vi "06_dosing.vi"() -> ()   [LabVIEW 2024]
uses:
  <vilib>/Utility/error.llb/DialogType.ctl
  7567123a-d5c5-487a-bc91-47e086c159d1.vi
  <vilib>/Waveform/WDTOps.llb/WDT Waveform to XY Pairs DBL.vi
  <instrlib>/Tektronix DMM40x0 Series/Tektronix DMM40x0 Series.lvlib
panel:
  out "Numeric":i32
  out "Waveform Graph 2":dbl[](array[numeric])
  out "STABLE":bool
  in  "Serial Communication":T1={"Baud Rate"=9600, "Parity"=0, "Data Bits"=8, "Stop Bits"=10, "Flow Control"=0} {"Flow Control" items=["None", "XON/XOFF", "RTS/CTS", "XON/XOFF & RTS/CTS", "DTR/DSR", "XON/XOFF & DTR/DSR"]; "Stop Bits" items=["1.0"=10, "1.5"=15, "2.0"=20]; "Data Bits" items=["7"=7, "8"=8]; "Parity" items=["None", "Odd", "Even", "Mark", "Space"]; "Baud Rate" items=["300"=300, "600"=600, "1200"=1200, "2400"=2400, "4800"=4800, "9600"=9600, "19200"=19200]}
  in  "COM PORT (COM2)":refnum<visa-resource-name>
  out "Stability threshold":dbl format="%#_13g"
  out "Waveform Graph":dbl[](graph)
  # "Voltmeter Serial Configuration"
  # "DEFAULT SETTINGS:\n\nTimeout (10000 ms)\nTrigger Count (5000)\nSample Count (1)\n\n****DC VOLTAGE***"
  # "Voltmeter Stability"
  # "0 - Stability threshold not met\n1 - Stability threshold met\n\n\n\n*stability (+/-0.05 mV) of last 15 pts"
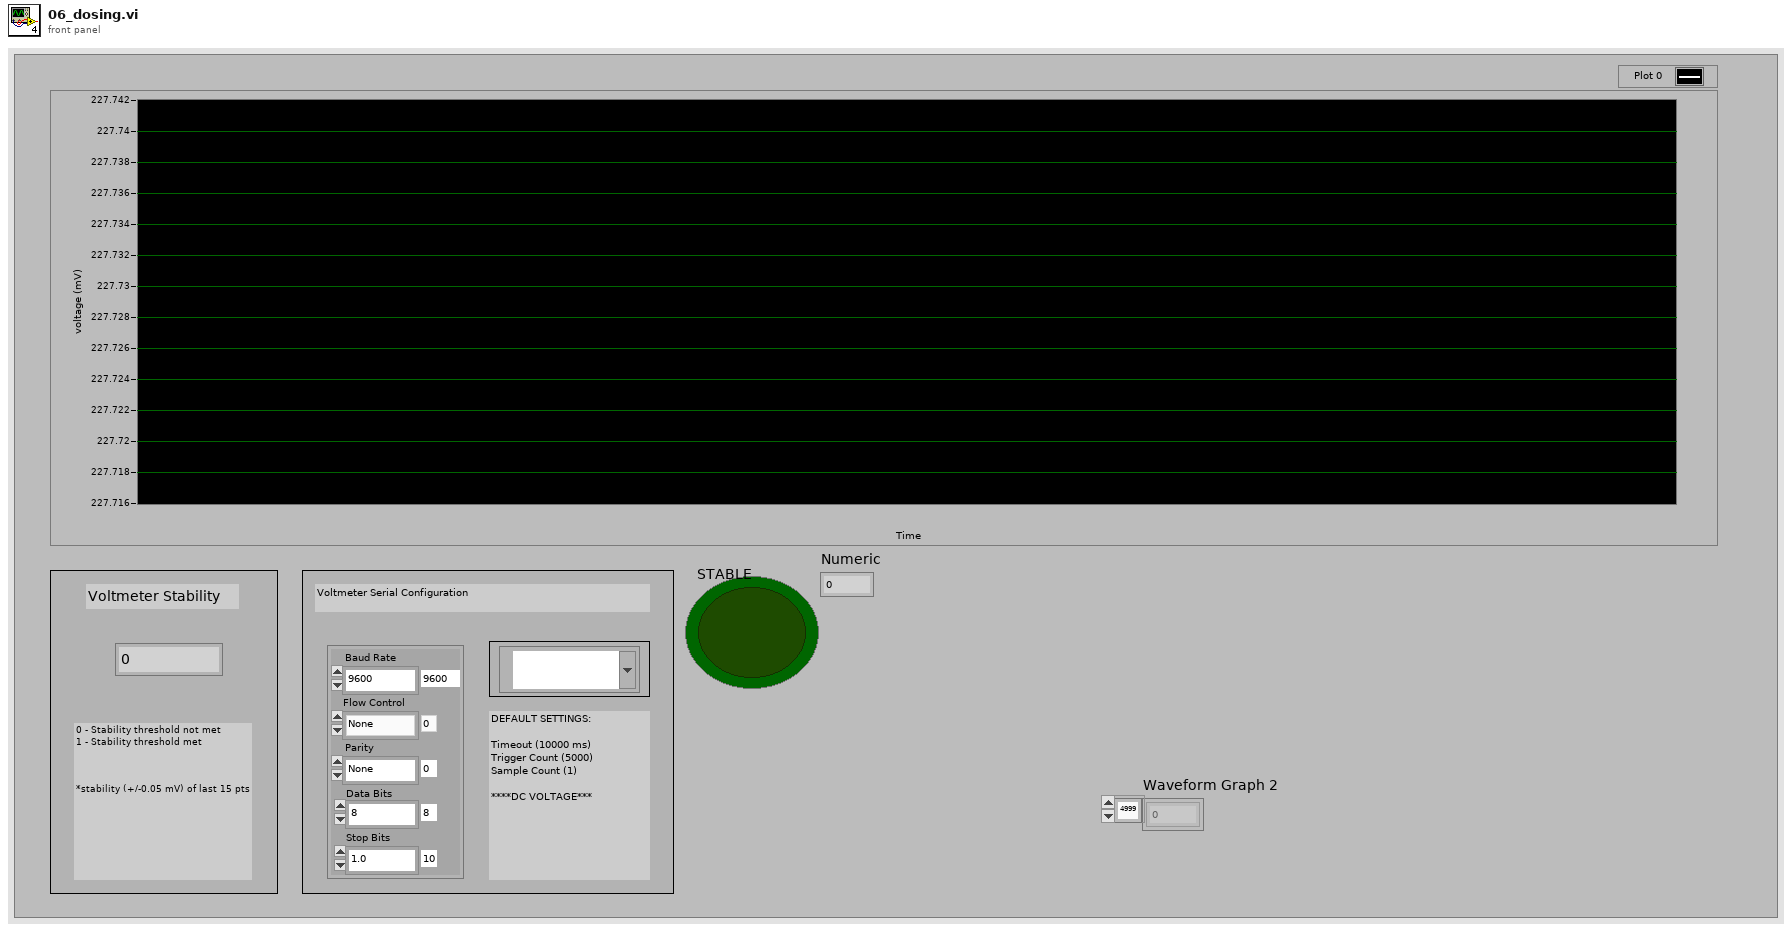
[diagram p1: front panel]
types:
  T1 = cluster{"Baud Rate":u32, "Parity":u16, "Data Bits":u16, "Stop Bits":u16, "Flow Control":u16}
  T2 = typedef "DialogType.ctl" = u16
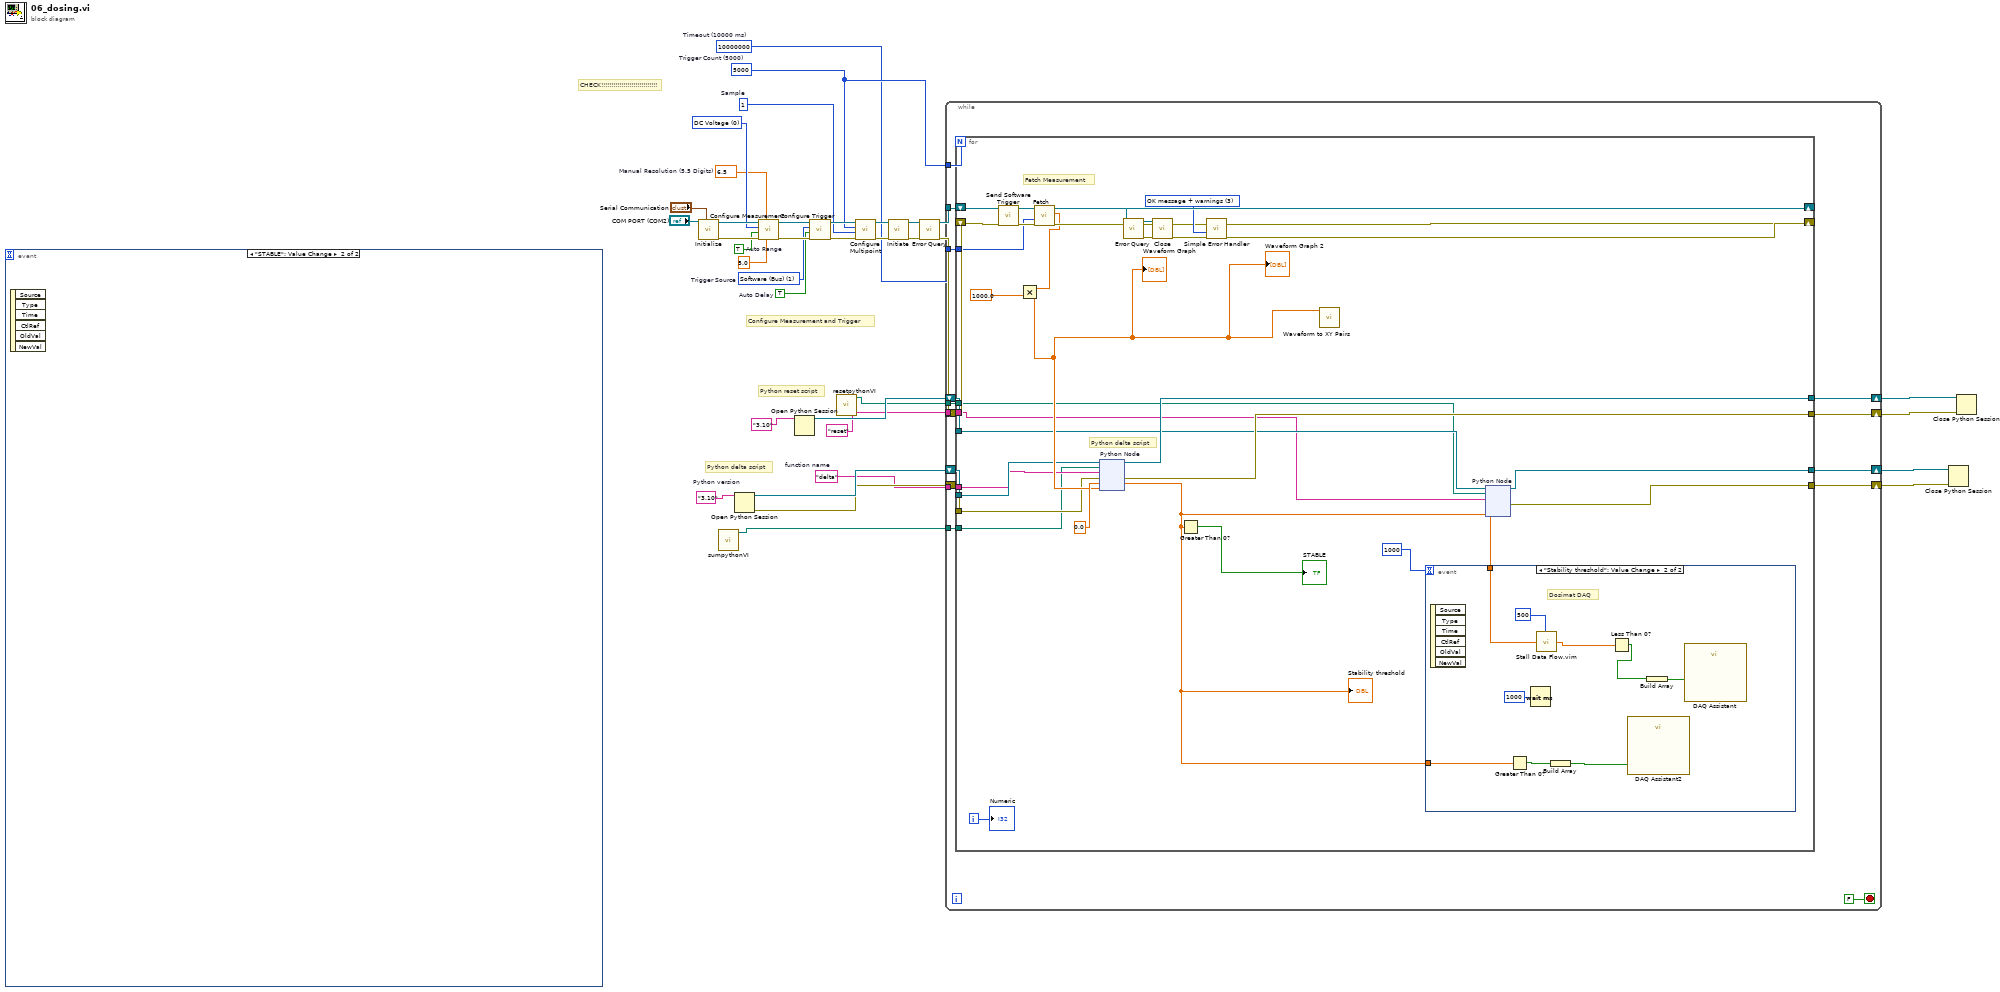
[diagram p0: block diagram]
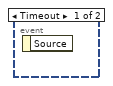
[diagram p2: hidden frame]
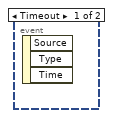
[diagram p3: hidden frame]
diagram:
  w8 = "delta"  # function name
  w11 = "3.10"  # Python version
  w23 = u16 0 items=["DC Voltage", "AC Voltage", "2 - Wire Resistance", "4 - Wire Resistance", "DC Current", "AC Current", "Frequency", "Period", "Continuity", "Diode Checking", "Temperature", "Capacitance"] ("Function (0: DC Voltage)")
  w14 = u32 10000000  # Timeout (10000 ms)
  w15 = 1  # Sample
  w22 = 5000  # Trigger Count (5000)
  w16 = 6.5 items=["4.5"=4.5, "5.5"=5.5, "6.5"=6.5]  # Manual Resolution (5.5 Digits)
  w24 = TRUE  # Auto Delay
  w25 = u16 1 items=["Immediate", "Software (Bus)", "External"]  # Trigger Source
  w26 = TRUE  # Auto Range
  # "Python delta script"
  # "Python reset script"
  # "CHECK!!!!!!!!!!!!!!!!!!!!!!!!!!!!"
  # "Configure Measurement and Trigger"
  n1 = event shown="[1] \"STABLE\": Value Change" {
    selector: _ -> [_ _]
    dyn-events: _ -> [_ _]
    timeout: _ -> [_ _]
    event Timeout {
      n2 = event-data() -> ()  [unwired: 1 in, 3 out]
    }
    event "STABLE": Value Change {
      n3 = event-data() -> ()  [unwired: 1 in, 6 out]
    }
  }
  n4 = call <instrlib>:"Initialize.vi"("Serial Configuration"="Serial Communication", "VISA resource name"="COM PORT (COM2)") -> ("error out"=w35:errorcluster, "VISA resource name out"=w36:refnum<visa-resource-name>)  [unwired: 3 in, 5 out]
  n5 = call "sumpythonVI.vi"() -> ("appended path"=w1:path)  [unwired: 11 in]
  n6 = Open Python Session(python version=w11) -> (session out=w13:refnum<k35>, error out=w12:errorcluster)  [unwired: 2 in]
  n7 = call <instrlib>:"Configure Measurement.vi"("Manual Range (1.0)"=5.0, "Manual Resolution (5.5 Digits)"=w16, "error in (no error)"=w35, "Auto Range (T:Enable)"=w26, "Function (0: DC Voltage)"=w23, "VISA resource name"=w36) -> ("error out"=w33:errorcluster, "VISA resource name out"=w34:refnum<visa-resource-name>)  [unwired: 4 out]
  n8 = Open Python Session(python version="3.10" ("Python version")) -> (session out=w9:refnum<k35>)  [unwired: 2 in, 1 out]
  n9 = call <instrlib>:"Configure Trigger.vi"("error in (no error)"=w33, "Auto Delay (T: Enable)"=w24, "Trigger Source (0: Immediate)"=w25, "VISA resource name"=w34) -> ("error out"=w31:errorcluster, "VISA resource name out"=w32:refnum<visa-resource-name>)  [unwired: 1 in, 5 out]
  n10 = call "resetpythonVI.vi"() -> ("appended path"=w7:path)  [unwired: 11 in]
  n11 = call <instrlib>:"Configure Multipoint.vi"("error in (no error)"=w31, "Sample Count (1)"=w15, "Trigger Count (1)"=w22, "VISA resource name"=w32) -> ("error out"=w29:errorcluster, "VISA resource name out"=w30:refnum<visa-resource-name>)  [unwired: 6 out]
  n12 = call <instrlib>:"Initiate.vi"("error in (no error)"=w29, "VISA resource name"=w30) -> ("error out"=w21:errorcluster, "VISA resource name out"=w20:refnum<visa-resource-name>)  [unwired: 8 out]
  n13 = call <instrlib>:"Error Query.vi"("error in (no error)"=w21, "VISA resource name"=w20) -> ("error out"=w18:errorcluster, "VISA resource name out"=w19:refnum<visa-resource-name>)  [unwired: 8 out]
  n14 = while {
    tunnel: w22 -> [w52]
    tunnel: w19 -> [w51]
    tunnel: w14 -> [w49]
    tunnel: w8 -> [w45]
    tunnel: w7 -> [w44]
    tunnel: "reset" ("function name") -> [w43]
    tunnel: w1 -> [w38]
    shift-right: [w39] -> w2
    shift-left: w18 -> [w50]
    shift-right: [w42] -> w5
    shift-left: w13 -> [w48]
    shift-right: [w41] -> w4
    shift-left: w12 -> [w47]
    shift-right: [w40] -> w3
    shift-left: w9 -> [w46]
    stop <- FALSE stop-if-true
    w53 = T2 3 items=["no dialog", "OK message", "continue or stop message", "OK message + warnings", "continue/stop + warnings"] ("type of dialog (OK msg:1)")
    n15 = for {
      N: w52 -> [_]
      shift-right: [w84] -> w55
      shift-left: w50 -> [w80]
      shift-right: [w85] -> w57
      shift-left: w51 -> [w81]
      tunnel: w49 -> [w79]
      tunnel: w48 -> [w73]
      tunnel: w47 -> [w72]
      tunnel: w46 -> [w65]
      tunnel: w45 -> [w71]
      tunnel: w38 -> [w70]
      tunnel: w44 -> [w64]
      tunnel: w43 -> [w63]
      tunnel: [w62] -> w42
      tunnel: [w61] -> w41
      tunnel: [w69] -> w40
      tunnel: [w68] -> w39
      i -> [w59]
      # "Python delta script"
      # "Fetch Measurement"
      n16 = call <instrlib>:"Send Software Trigger.vi"("error in (no error)"=w80, "VISA resource name"=w81) -> ("error out"=w82:errorcluster, "VISA resource name out"=w83:refnum<visa-resource-name>)  [unwired: 8 out]
      n17 = call <instrlib>:"Fetch.vi"("error in (no error)"=w82, "Timeout (10000 ms)"=w79, "VISA resource name"=w83) -> ("error out"=w84:errorcluster, "Measurements"=w77:dbl[], "VISA resource name out"=w85:refnum<visa-resource-name>)  [unwired: 6 out]
      n18 = Multiply(x=w77, y=1000.0) -> (x*y=w76:dbl[])
      "Waveform Graph" <- w76
      "Waveform Graph 2" <- w76
      n19 = node "Python Node"(w73, w70, w71, w72, 0.0, w76) -> (w69:refnum<k35>, w68:errorcluster, w66:dbl)  [unwired: 1 in, 2 out]
      "Stability threshold" <- w66
      n20 = Greater Than 0?(x=w66) -> (x > 0?=→"STABLE":bool)
      n21 = call-poly <vilib>:"Waveform to XY Pairs.vi"("waveform in"=w76) -> ()  [unwired: 8 in, 3 out]
      n22 = node "Python Node"(w65, w64, w63, w66) -> (w62:refnum<k35>, w61:errorcluster, w60:dbl)  [unwired: 3 in, 2 out]
      n23 = event shown="[1] \"Stability threshold\": Value Change" {
        selector: _ -> [_ _]
        dyn-events: _ -> [_ _]
        timeout: 1000 -> [_ _]
        tunnel: w66 -> [_ w87]
        tunnel: w60 -> [_ w86]
        event Timeout {
          n24 = event-data() -> ()  [unwired: 1 in, 1 out]
        }
        event "Stability threshold": Value Change {
          # "Dosimat DAQ"
          n25 = event-data() -> ()  [unwired: 1 in, 6 out]
          n26 = Greater Than 0?(x=w87) -> (x > 0?=w92:bool)
          n27 = Wait (ms)(milliseconds to wait=u32 1000) -> ()  [unwired: 1 out]
          n28 = call "Stall Data Flow.vim"("value in"=w86, "milliseconds to wait"=u32 500) -> ("value out"=w90:dbl)  [unwired: 1 out]
          n29 = Build Array(w92) -> (w91:bool[])
          n30 = Less Than 0?(x=w90) -> (x < 0?=w93:bool)
          n31 = call "DAQ Assistant2"("data"=w91) -> ()  [unwired: 17 in, 2 out]
          n32 = Build Array(w93) -> (w94:bool[])
          n33 = call "DAQ Assistant"("data"=w94) -> ()  [unwired: 17 in, 2 out]
        }
      }
      "Numeric" <- w59
    }
    n34 = call <instrlib>:"Error Query.vi"("error in (no error)"=w55, "VISA resource name"=w57) -> ("error out"=w54:errorcluster, "VISA resource name out"=w56:refnum<visa-resource-name>)  [unwired: 8 out]
    n35 = call <instrlib>:"Close.vi"("error in (no error)"=w54, "VISA resource name"=w56) -> ("error out"=w58:errorcluster)  [unwired: 9 out]
    n36 = call <vilib>:"Simple Error Handler.vi"("type of dialog (OK msg:1)"=w53, "error in (no error)"=w58) -> ()  [unwired: 8 out]
  }
  n37 = Close Python Session(session in=w5, error in=w4) -> ()  [unwired: 1 out]
  n38 = Close Python Session(session in=w3, error in=w2) -> ()  [unwired: 1 out]
